vi "Write Banks.vi"(8 "error in (no error)":errorcluster, 10 "Ports":u8[](array[numeric]), 11 "DIG_IO in":refnum<class "DIG_IO.lvclass">) -> (0 "error out":errorcluster, 3 "DIG_IO out":refnum<class "DIG_IO.lvclass">)   [LabVIEW 2019, in "DIG_IO.lvlib" / "DIG_IO.lvclass"]
uses:
  Library/DIG_IO.lvclass
  Library/DIG_IO.lvclass/DIG_IO.ctl
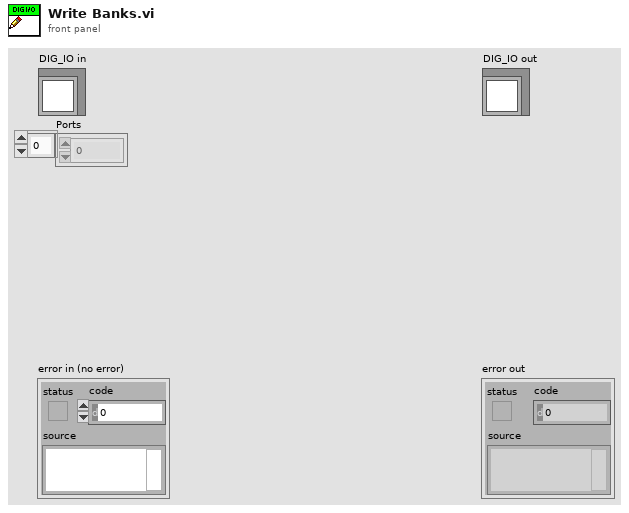
[diagram p1: front panel]
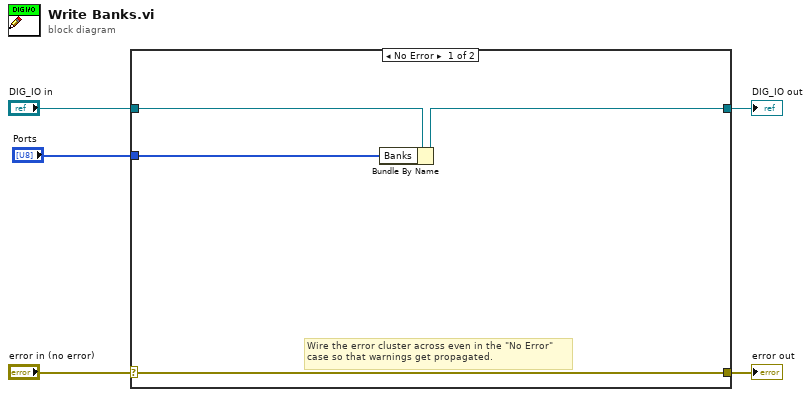
[diagram p0: block diagram]
diagram:
  n1 = case shown="No Error" "error in (no error)" {
    selector: "error in (no error)" -> [w8 w11]
    tunnel: [w8 w11] -> w4
    tunnel: [w7 w10] -> w2
    tunnel: "DIG_IO in" -> [w9 w10]
    tunnel: "Ports" -> [w6 _]
    frame No Error {
      # "Wire the error cluster across even in the \"No Error\"\ncase so that warnings get propagated."
      n2 = Bundle By Name(cluster=w9, "Banks"=w6) -> (w7:refnum<class "DIG_IO.lvclass">)
    }
    frame Error {
    }
  }
  "error out" <- w4
  "DIG_IO out" <- w2
